vi "Read Analogue.vi"(8 "error in (no error)":errorcluster, 11 "Lambda Gen LAN in":refnum<class "Lambda Gen LAN.lvclass">) -> (0 "error out":errorcluster, 2 "Waveforms":waveform(dbl)[](array[waveform]), 3 "Lambda Gen LAN out":refnum<class "Lambda Gen LAN.lvclass">)   [LabVIEW 2025, in "Power Supply.lvlib" / "Lambda Gen LAN.lvclass"]
uses:
  Lambda Gen LAN.lvclass
  C:/Users/Public/Documents/Sandia National Labs/TSS Plugin/Abstract Engine.lvlibp/Abstract Instrument/Abstract Instrument.lvclass
  Lambda Gen LAN.lvclass/Lambda Gen LAN.ctl
  <instrlib>/TDK-Lambda GEN LAN Series/TDK-Lambda GEN LAN Series.lvlib
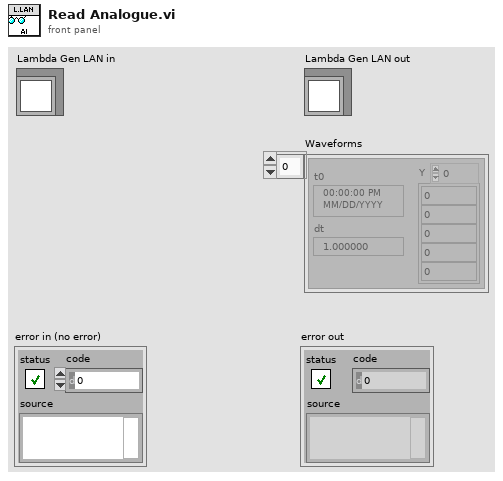
[diagram p1: front panel]
types:
  T1 = typedef "Abstract Engine.lvlibp/Abstract Instrument.lvclass/Channel.ctl" = cluster{"Alias":string, "DataType":enum16{"Anaolg Input", "Waveform"}, "Unit":enum16{"---", "V", "A", "Ohm", "Hz", "uF", "degC", "deg"}, "Upper limit":dbl, "Lower limit":dbl, "Measurement":variant}
  T2 = cluster{"Output Voltage":dbl, "Output Current":dbl}
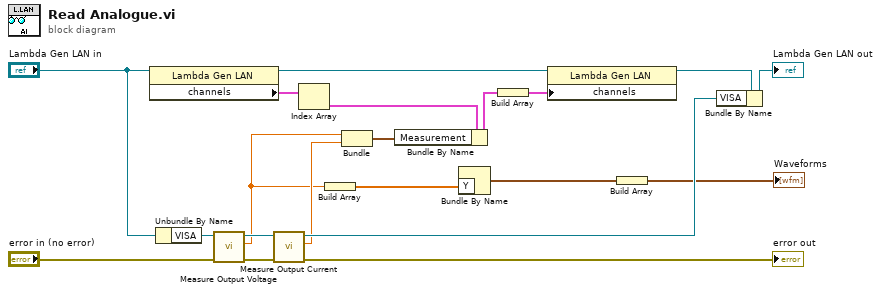
[diagram p0: block diagram]
diagram:
  n1 = property class="Lambda Gen LAN"(reference="Lambda Gen LAN in") -> (reference out=w11:refnum<class "Lambda Gen LAN.lvclass">, "channels"=w10:T1[])  [unwired: 1 in, 1 out]
  n2 = Unbundle By Name("Lambda Gen LAN in") -> ("VISA"=w19:refnum<visa-resource-name>)
  n3 = call <instrlib>:"Measure Output Voltage.vi"("error"="error in (no error)", "VISA"=w19) -> ("error out"=w16:errorcluster, "Output Voltage"=w4:dbl, "VISA out"=w14:refnum<visa-resource-name>)  [unwired: 7 in]
  n4 = call <instrlib>:"Measure Output Current.vi"("error"=w16, "VISA"=w14) -> ("error out"=→"error out":errorcluster, "Output Current"=w8:dbl, "VISA out"=w12:refnum<visa-resource-name>)  [unwired: 7 in]
  n5 = Index Array(array=w10) -> (element=w5:T1)  [unwired: 1 in]
  n6 = Build Array(w4) -> (w3:dbl[])
  n7 = Bundle("Output Voltage"=w4, "Output Current"=w8) -> (w9:T2)  [unwired: 1 in]
  n8 = Bundle By Name(cluster=w5, "Measurement"=w9) -> (w6:T1)
  n9 = Bundle By Name("Y"=w3) -> (w2:waveform(dbl))  [unwired: 1 in]
  n10 = Build Array(w6) -> (w7:T1[])
  n11 = property class="Lambda Gen LAN"(reference=w11, "channels"=w7) -> (reference out=w17:refnum<class "Lambda Gen LAN.lvclass">)  [unwired: 1 in, 1 out]
  n12 = Build Array(w2) -> (→"Waveforms":waveform(dbl)[])
  n13 = Bundle By Name(cluster=w17, "VISA"=w12) -> (→"Lambda Gen LAN out":refnum<class "Lambda Gen LAN.lvclass">)
